vi "pathplan.vi"(8 "当前位置":dbl[](array[numeric]), 9 "目标位置（x,y）":dbl[](array[numeric]), 10 "障碍物Y":dbl[](array[numeric]), 11 "障碍物X":dbl[](array[numeric])) -> (1 "y":dbl[](array[numeric]), 2 "x":dbl[](array[numeric]))   [LabVIEW 2016]
uses:
  <vilib>/gmath/SpecialFunctions.llb/Factorial.vi
  <vilib>/imath/engines/lvmath2/RunTimeEngine/BuiltInFunctions/size/NIMS_I32Row=size(GRow).vi
  <instcachedir>/0/NIMS_I32Row=size(GRow)_E5C05C6B13124B29B774CC4F993D3C59.lvgen/NIMS_I32Row=size(GRow)_E5C05C6B13124B29B774CC4F993D3C59_000.vi
  <vilib>/imath/engines/lvmath2/RunTimeEngine/IndexRead/NIMS M(S,S).vi
  <instcachedir>/0/NIMS M(S,S)_AC51E74150A542F7991B9634C66F3096.lvgen/NIMS M(S,S)_AC51E74150A542F7991B9634C66F3096_002.vi
  <vilib>/imathl/engines/lvmath/Functions/Error Handling/Create Error.vi
  <vilib>/imath/engines/lvmath2/RunTimeEngine/IndexRead/NIMS V(S).vi
  <instcachedir>/0/NIMS V(S)_0488751826AF41519A22953C041130DC.lvgen/NIMS V(S)_0488751826AF41519A22953C041130DC_000.vi
  <vilib>/imath/engines/lvmath2/RunTimeEngine/IndexReplace/NIMS V(S)=S.vi
  <instcachedir>/0/NIMS V(S)=S_5B9D821375184D3582A2146CD1A04ED7.lvgen/NIMS V(S)=S_5B9D821375184D3582A2146CD1A04ED7_001.vi
  <vilib>/imath/engines/lvmath2/RunTimeEngine/ErrorHandling/NIMS_Create Error From Enums.vi
  <vilib>/imath/engines/lvmath2/RunTimeEngine/BuiltInFunctions/power/NIMS_power.vi
  <instcachedir>/0/NIMS_power_10DB0E02FC3E47EE88A20FD73927AD27.lvgen/NIMS_power_10DB0E02FC3E47EE88A20FD73927AD27_016.vi
  <instcachedir>/0/NIMS V(S)_0488751826AF41519A22953C041130DC.lvgen/NIMS V(S)_0488751826AF41519A22953C041130DC_003.vi
  <vilib>/imath/engines/lvmath2/RunTimeEngine/BuiltInFunctions/cos/NIMS_cos(C).vi
  <instcachedir>/0/NIMS_cos(C)_6CBFAE4528E34B94A77DA2891B495EBE.lvgen/NIMS_cos(C)_6CBFAE4528E34B94A77DA2891B495EBE_001.vi
  <vilib>/imath/engines/lvmath2/RunTimeEngine/BuiltInFunctions/abs/NIMS_abs(signed).vi
  <instcachedir>/0/NIMS_abs(signed)_C4FCB8E6058B49B797C7C8D53CA5F6EC.lvgen/NIMS_abs(signed)_C4FCB8E6058B49B797C7C8D53CA5F6EC_002.vi
  <vilib>/imath/engines/lvmath2/RunTimeEngine/RangeToken/NIMS_Range_R2 - Integer.vi
  <instcachedir>/0/NIMS_Range_R2 - Integer_416A044C4F024DBE8E97DA138CB3186F.lvgen/NIMS_Range_R2 - Integer_416A044C4F024DBE8E97DA138CB3186F_000.vi
  <vilib>/imath/engines/lvmath2/RunTimeEngine/CommandStatement/MC_CommandStatement_break.vi
  <vilib>/imath/engines/lvmath/Functions/Error Handling/MergeErrorsWrapper.vi
  <vilib>/imath/engines/lvmath2/RunTimeEngine/IndexReplace/NIMS M(S)=S.vi
  <instcachedir>/0/NIMS M(S)=S_9328EF344EC9443A8B5E4239F1A18A91.lvgen/NIMS M(S)=S_9328EF344EC9443A8B5E4239F1A18A91_001.vi
  <vilib>/imath/engines/lvmath2/RunTimeEngine/ArithmeticOperatorToken/NIMS_ArithmeticOperator_minus.vi
  <instcachedir>/0/NIMS_ArithmeticOperator_minus_DDDC508CE2F847AF862BE7DD2E3133BB.lvgen/NIMS_ArithmeticOperator_minus_DDDC508CE2F847AF862BE7DD2E3133BB_003.vi
  <vilib>/imath/engines/lvmath2/RunTimeEngine/BuiltInFunctions/norm/NIMS_norm(GV,DBL).vi
  <instcachedir>/0/NIMS_norm(GV,DBL)_AEE3258AE133461381C802EA81F1ACD5.lvgen/NIMS_norm(GV,DBL)_AEE3258AE133461381C802EA81F1ACD5_000.vi
  <vilib>/imath/engines/lvmath2/RunTimeEngine/IndexRead/NIMS M(S).vi
  <instcachedir>/0/NIMS M(S)_B826C018497E4940AE96BD27B540B6FB.lvgen/NIMS M(S)_B826C018497E4940AE96BD27B540B6FB_000.vi
  <vilib>/imath/engines/lvmath2/RunTimeEngine/IndexRead/NIMS V(V).vi
  <instcachedir>/0/NIMS V(V)_298D9CB7BFEB42B8BC8D9C3C28AE8C70.lvgen/NIMS V(V)_298D9CB7BFEB42B8BC8D9C3C28AE8C70_000.vi
  <vilib>/imath/engines/lvmath2/RunTimeSupport/NIMS_Get Scalar_w Error.vi
  <instcachedir>/0/NIMS_Get Scalar_w Error_B10CD3EFE684481FAA3AC86F54EE16C9.lvgen/NIMS_Get Scalar_w Error_B10CD3EFE684481FAA3AC86F54EE16C9_010.vi
  <vilib>/imath/engines/lvmath2/RunTimeEngine/MatrixToken/NIMS_MatrixToken_RV_RV.vi
  <instcachedir>/0/NIMS_MatrixToken_RV_RV_EF9D95F1EBB54EC7B599CEAAF2A767A1.lvgen/NIMS_MatrixToken_RV_RV_EF9D95F1EBB54EC7B599CEAAF2A767A1_002.vi
  <vilib>/imath/engines/lvmath2/RunTimeEngine/MatrixToken/NIMS_MatrixToken_M_RV.vi
  <instcachedir>/0/NIMS_MatrixToken_M_RV_FA7C223A39F54BCB827124D804A50E22.lvgen/NIMS_MatrixToken_M_RV_FA7C223A39F54BCB827124D804A50E22_001.vi
  <vilib>/imath/engines/lvmath2/RunTimeEngine/BuiltInFunctions/max/2 inputs/NIMS_max(RG,RG)-no size check.vi
  <instcachedir>/0/NIMS_max(RG,RG)-no size check_F871939977644B7683C1350DCCAD7557.lvgen/NIMS_max(RG,RG)-no size check_F871939977644B7683C1350DCCAD7557_000.vi
  <instcachedir>/0/NIMS M(S,S)_AC51E74150A542F7991B9634C66F3096.lvgen/NIMS M(S,S)_AC51E74150A542F7991B9634C66F3096_000.vi
  <vilib>/imath/engines/lvmath2/RunTimeEngine/BuiltInFunctions/min/2 inputs/NIMS_min(RG,RG)-no size check.vi
  <instcachedir>/0/NIMS_min(RG,RG)-no size check_7F67BAB91AFC452D9517D2EA1C8F5F88.lvgen/NIMS_min(RG,RG)-no size check_7F67BAB91AFC452D9517D2EA1C8F5F88_001.vi
  <instcachedir>/0/NIMS_abs(signed)_C4FCB8E6058B49B797C7C8D53CA5F6EC.lvgen/NIMS_abs(signed)_C4FCB8E6058B49B797C7C8D53CA5F6EC_000.vi
  <vilib>/imath/engines/lvmath2/RunTimeEngine/VariableToken/NIMS_VariableToken_CondDefined.vi
  <instcachedir>/0/NIMS_VariableToken_CondDefined_620A15720FCC4DA7863546285C12295E.lvgen/NIMS_VariableToken_CondDefined_620A15720FCC4DA7863546285C12295E_001.vi
  <vilib>/imath/engines/lvmath2/RunTimeEngine/BuiltInFunctions/size/NIMS_I32=size(GM,I32).vi
  <instcachedir>/0/NIMS_I32=size(GM,I32)_9B6975FE2A37478D9DF1A6A9597B9E6B.lvgen/NIMS_I32=size(GM,I32)_9B6975FE2A37478D9DF1A6A9597B9E6B_004.vi
  <vilib>/imath/engines/lvmath2/RunTimeEngine/NodeEndStatement/NIMS_NodeEndStatement_Output.vi
  <instcachedir>/0/NIMS_NodeEndStatement_Output_53EC0D466D134D7ABD903AC30B43404B.lvgen/NIMS_NodeEndStatement_Output_53EC0D466D134D7ABD903AC30B43404B_005.vi
  <vilib>/imath/engines/lvmath2/RunTimeEngine/ErrorHandling/NIMS_Finalize Error.vi
  <vilib>/gmath/NI_Gmath.lvlib
panel:
  out "?":cluster{"Data_x":dbl[], "Data_y":dbl[]}(graph)
  out "x/y":dbl[](array[numeric])
  out "?":cluster{"Data_x":dbl[], "Data_y":dbl[]}(graph)
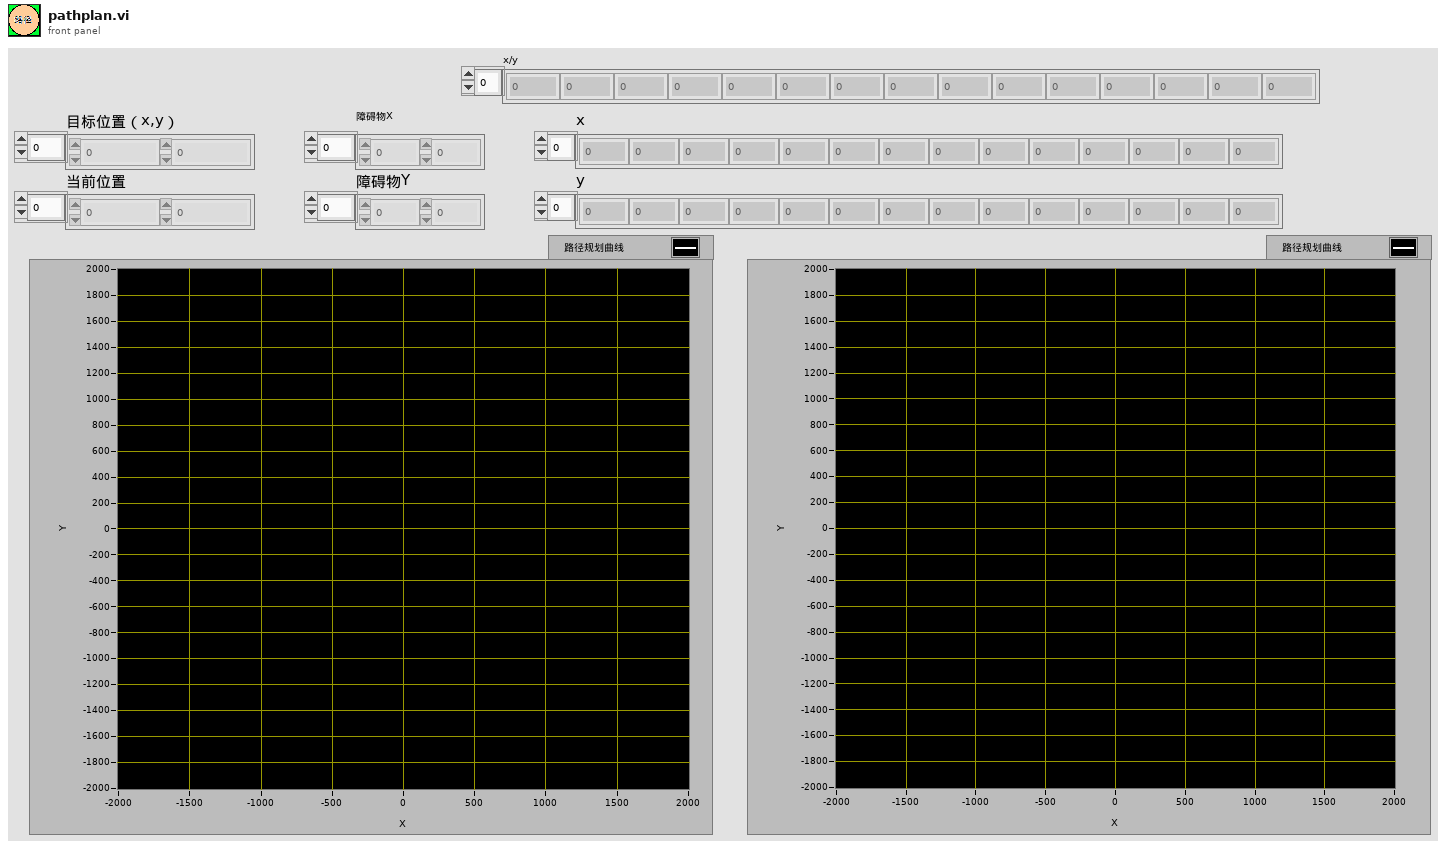
[diagram p1: front panel]
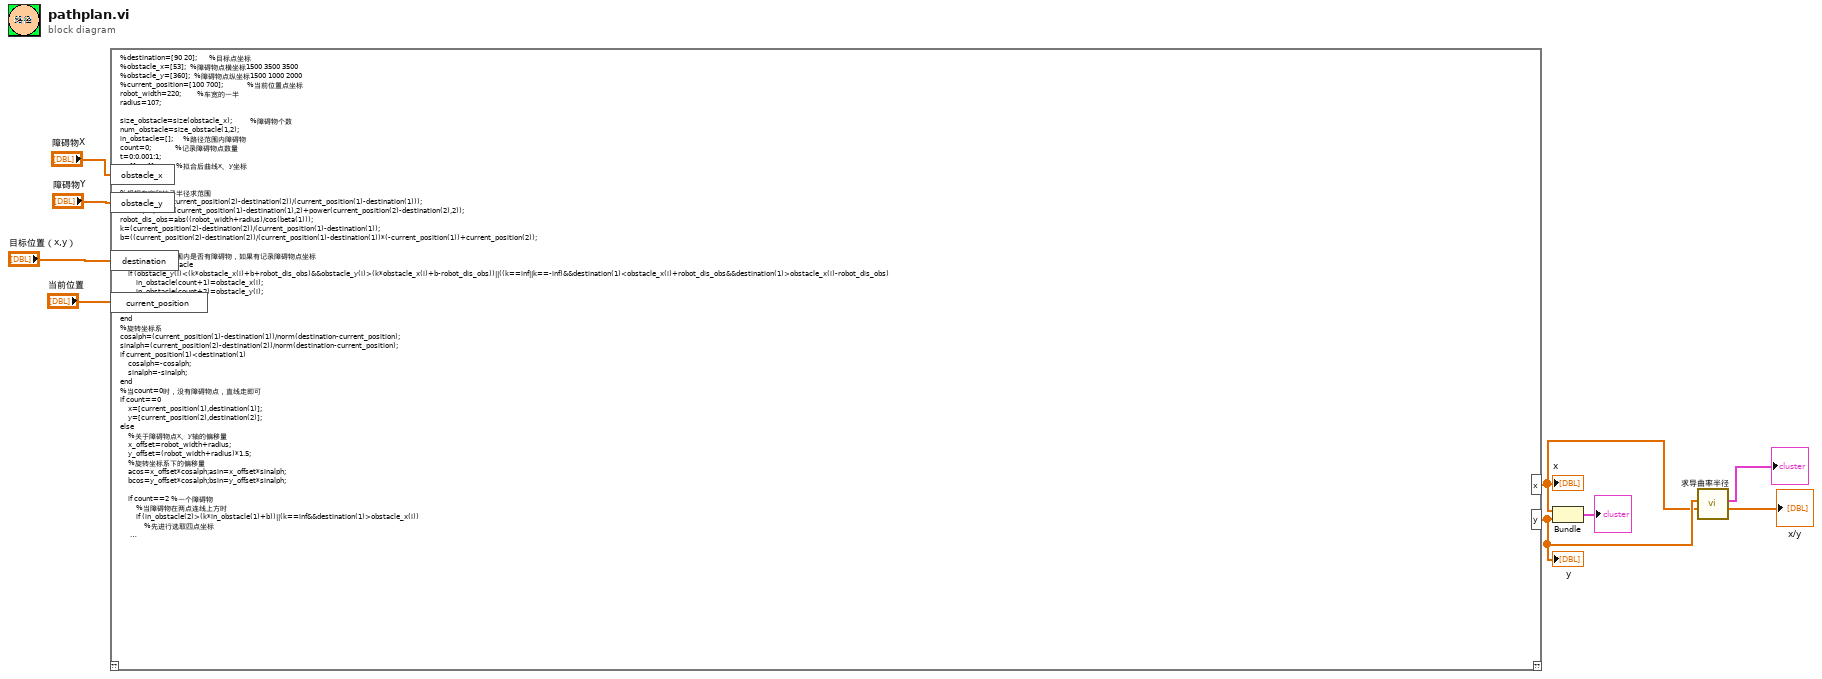
[diagram p0: block diagram]
diagram:
  n1 = mathscript code="%destination=[90 20];      %目标点坐标\n%obstacle_x=[53];  %障碍物点横坐标1500 3500 3500\n%obstacle_y=[360];  %障碍物点纵坐标1500 1000 2000\n%current_position=[100 700];            %当前位置点坐标\nrobot_width=220;        %车宽的一半\nradius=107;\n\nsize_obstacle=size(obstacle_x);         %障碍物个数\nnum_obstacle=size_obstacle(1,2);\nin_obstacle=[];     %路径范围内障碍物\ncount=0;            %记录障碍物点数量\nt=0:0.001:1;\nx=[];y=[];          %拟合后曲线x、y坐标\n\n\n%根据车宽和柱子半径求范围\nbeta(1)=atan((current_position(2)-destination(2))/(current_position(1)-destination(1)));\ndis=sqrt(power(current_position(1)-destination(1),2)+power(current_position(2)-destination(2),2));\nrobot_dis_obs=abs((robot_width+radius)/cos(beta(1)));\nk=(current_position(2)-destination(2))/(current_position(1)-destination(1));\nb=((current_position(2)-destination(2))/(current_position(1)-destination(1))*(-current_position(1))+current_position(2));\n\n%判断直行路径范围内是否有障碍物，如果有记录障碍物点坐标\nfor i=1:num_obstacle\n    if (obstacle_y(i)<(k*obstacle_x(i)+b+robot_dis_obs)&&obstacle_y(i)>(k*obstacle_x(i)+b-robot_dis_obs))||((k==inf||k==-inf)&&destination(1)<obstacle_x(i)+robot_dis_obs&&destination(1)>obstacle_x(i)-robot_dis_obs)\n        in_obstacle(count+1)=obstacle_x(i);\n        in_obstacle(count+2)=obstacle_y(i);\n        count=count+2;\n    end\nend\n%旋转坐标系\ncosalph=(current_position(1)-destination(1))/norm(destination-current_position);\nsinalph=(current_position(2)-destination(2))/norm(destination-current_position);\nif current_position(1)<destination(1)\n    cosalph=-cosalph;\n    sinalph=-sinalph;\nend\n%当count=0时，没有障碍物点，直线走即可\nif count==0\n    x=[current_position(1),destination(1)];\n    y=[current_position(2),destination(2)];\nelse\n    %关于障碍物点x、y轴的偏移量\n    x_offset=robot_width+radius;\n    y_offset=(robot_width+radius)*1.5;\n    %旋转坐标系下的偏移量\n    acos=x_offset*cosalph;asin=x_offset*sinalph;\n    bcos=y_offset*cosalph;bsin=y_offset*sinalph;\n    \n    if count==2 %一个障碍物\n        %当障碍物在两点连线上方时\n        if (in_obstacle(2)>(k*in_obstacle(1)+b))||(k==inf&&destination(1)>obstacle_x(i))\n            %先进行选取四点坐标\n            temp_position1=[in_obstacle(1)+acos+bsin,in_obstacle(2)+asin-bcos];\n            temp_position2=[in_obstacle(1)-acos+bsin,in_obstacle(2)-asin-bcos];\n            if current_position(1)>destination(1)\n                if temp_position1(1)>temp_position2(1)\n                    vertices=[current_position;temp_position1;temp_position2;destination]';\n                else\n                    vertices=[current_position;temp_position2;temp_position1;destination]';\n                end\n            else\n                if temp_position1(1)>temp_position2(1)\n                    vertices=[current_position;temp_position2;temp_position1;destination]';\n                else\n                    vertices=[current_position;temp_position1;temp_position2;destination]';\n                end\n            end\n            %检测两两坐标连线上是否会遇到障碍物\n            for i=1:num_obstacle\n                %待检测出的障碍物的横坐标应不等于已检测出障碍物点的横坐标，检测右边是否有障碍物\n                if (obstacle_x(i)~=in_obstacle(1))&&(obstacle_x(i)<max(current_position(1),destination(1)))&&(obstacle_y(i)<((vertices(2,2)-vertices(2,1))/(vertices(1,2)-vertices(1,1))*obstacle_x(i)+vertices(2,2)-(vertices(2,2)-vertices(2,1))/(vertices(1,2)-vertices(1,1))*vertices(1,2)+robot_dis_obs))&&(obstacle_y(i)>((vertices(2,2)-vertices(2,1))/(vertices(1,2)-vertices(1,1))*obstacle_x(i)+vertices(2,2)-(vertices(2,2)-vertices(2,1))/(vertices(1,2)-vertices(1,1))*vertices(1,2)-robot_dis_obs))\n                    in_obstacle(count+1)=obstacle_x(i);     %若有，记录下该障碍物点的横纵坐标，count加2\n                    in_obstacle(count+2)=obstacle_y(i);\n                    count=count+2;\n                    %检测左边是否有障碍物\n                elseif (obstacle_x(i)~=in_obstacle(1))&&(obstacle_x(i)>min(current_position(1),destination(1)))&&(obstacle_y(i)<((vertices(2,4)-vertices(2,3))/(vertices(1,4)-vertices(1,3))*obstacle_x(i)+vertices(2,4)-(vertices(2,4)-vertices(2,3))/(vertices(1,4)-vertices(1,3))*vertices(1,4)+robot_dis_obs))&&(obstacle_y(i)>((vertices(2,4)-vertices(2,3))/(vertices(1,4)-vertices(1,3))*obstacle_x(i)+vertices(2,4)-(vertices(2,4)-vertices(2,3))/(vertices(1,4)-vertices(1,3))*vertices(1,4)-robot_dis_obs))\n                    tempx=in_obstacle(1);\n                    tempy=in_obstacle(2);\n                    in_obstacle(1)=obstacle_x(i);\n                    in_obstacle(2)=obstacle_y(i);\n                    in_obstacle(3)=tempx;\n                    in_obstacle(4)=tempy;\n                    count=count+2;\n                end\n            end\n        else\n            temp_position1=[in_obstacle(1)+acos-bsin,in_obstacle(2)+asin+bcos];\n            temp_position2=[in_obstacle(1)-acos-bsin,in_obstacle(2)-asin+bcos];\n            if current_position(1)>destination(1)\n                if temp_position1(1)>temp_position2(1)\n                    vertices=[current_position;temp_position1;temp_position2;destination]';\n                else\n                    vertices=[current_position;temp_position2;temp_position1;destination]';\n                end\n            else\n                if temp_position1(1)>temp_position2(1)\n                    vertices=[current_position;temp_position2;temp_position1;destination]';\n                else\n                    vertices=[current_position;temp_position1;temp_position2;destination]';\n                end\n            end\n            for i=1:num_obstacle\n                if (obstacle_x(i)~=in_obstacle(1))&&(obstacle_x(i)<max(current_position(1),destination(1)))&&(obstacle_y(i)<((vertices(2,2)-vertices(2,1))/(vertices(1,2)-vertices(1,1))*obstacle_x(i)+vertices(2,2)-(vertices(2,2)-vertices(2,1))/(vertices(1,2)-vertices(1,1))*vertices(1,2)+robot_dis_obs))&&(obstacle_y(i)>((vertices(2,2)-vertices(2,1))/(vertices(1,2)-vertices(1,1))*obstacle_x(i)+vertices(2,2)-(vertices(2,2)-vertices(2,1))/(vertices(1,2)-vertices(1,1))*vertices(1,2)-robot_dis_obs))\n                    in_obstacle(count+1)=obstacle_x(i);\n                    in_obstacle(count+2)=obstacle_y(i);\n                    count=count+2;\n                    break;\n                elseif (obstacle_x(i)~=in_obstacle(1))&&(obstacle_x(i)>min(current_position(1),destination(1)))&&(obstacle_y(i)<((vertices(2,4)-vertices(2,3))/(vertices(1,4)-vertices(1,3))*obstacle_x(i)+vertices(2,4)-(vertices(2,4)-vertices(2,3))/(vertices(1,4)-vertices(1,3))*vertices(1,4)+robot_dis_obs))&&(obstacle_y(i)>((vertices(2,4)-vertices(2,3))/(vertices(1,4)-vertices(1,3))*obstacle_x(i)+vertices(2,4)-(vertices(2,4)-vertices(2,3))/(vertices(1,4)-vertices(1,3))*vertices(1,4)-robot_dis_obs))\n                    tempx=in_obstacle(1);\n                    tempy=in_obstacle(2);\n                    in_obstacle(1)=obstacle_x(i);\n                    in_obstacle(2)=obstacle_y(i);\n                    in_obstacle(3)=tempx;\n                    in_obstacle(4)=tempy;\n                    count=count+2;\n                    break;\n                end\n            end\n        end\n    end\n    if count==2\n    else\n        %当两个都在直线上方时\n        if (in_obstacle(2)>(k*in_obstacle(1)+b)||in_obstacle(2)==(k*in_obstacle(1)+b))&&(in_obstacle(4)>(k*in_obstacle(3)+b)||in_obstacle(4)==(k*in_obstacle(3)+b))\n            temp_position1=[in_obstacle(3)+acos+bsin,in_obstacle(4)+asin-bcos];\n            temp_position2=[in_obstacle(3)-acos+bsin,in_obstacle(4)-asin-bcos];\n            temp_position3=[in_obstacle(1)+acos+bsin,in_obstacle(2)+asin-bcos];\n            temp_position4=[in_obstacle(1)-acos+bsin,in_obstacle(2)-asin-bcos];\n            if abs(current_position(1)-in_obstacle(3))<abs(current_position(1)-in_obstacle(1))\n                if abs(current_position(1)-temp_position1(1))<abs(current_position(1)-temp_position2(1))\n                    temp1=temp_position1;\n                    temp2=temp_position2;\n                else\n                    temp1=temp_position2;\n                    temp2=temp_position1;\n                end\n                if abs(destination(1)-temp_position3(1))>abs(destination(1)-temp_position4(1))\n                    temp3=temp_position3;\n                    temp4=temp_position4;\n                else\n                    temp3=temp_position4;\n                    temp4=temp_position3;\n                end\n                vertices=[current_position;temp1;temp2;temp3;temp4;destination ]';\n            else\n                if abs(current_position(1)-temp_position3(1))<abs(current_position(1)-temp_position4(1))\n                    temp1=temp_position3;\n                    temp2=temp_position4;\n                else\n                    temp1=temp_position4;\n                    temp2=temp_position3;\n                end\n                if abs(destination(1)-temp_position1(1))>abs(destination(1)-temp_position2(1))\n                    temp3=temp_position1;\n                    temp4=temp_position2;\n                else\n                    temp3=temp_position2;\n                    temp4=temp_position1;\n                end\n                vertices=[current_position;temp1;temp2;temp3;temp4;destination ]';\n            end\n            %当右侧的在直线下方，左侧的在直线上方\n        elseif in_obstacle(2)<(k*in_obstacle(1)+b)&&in_obstacle(4)>(k*in_obstacle(3)+b)\n            y_offset=(robot_width+radius)*2;\n            bcos=y_offset*cosalph;bsin=y_offset*sinalph;\n            temp_position1=[in_obstacle(3)+acos+bsin,in_obstacle(4)+asin-bcos];\n            temp_position2=[in_obstacle(3)-acos+bsin,in_obstacle(4)-asin-bcos];\n            temp_position3=[in_obstacle(1)+acos-bsin,in_obstacle(2)+asin+bcos];\n            temp_position4=[in_obstacle(1)-acos-bsin,in_obstacle(2)-asin+bcos];\n            if abs(current_position(1)-in_obstacle(3))<abs(current_position(1)-in_obstacle(1))\n                if abs(current_position(1)-temp_position1(1))<abs(current_position(1)-temp_position2(1))\n                    temp1=temp_position1;\n                    temp2=temp_position2;\n                else\n                    temp1=temp_position2;\n                    temp2=temp_position1;\n                end\n                if abs(destination(1)-temp_position3(1))>abs(destination(1)-temp_position4(1))\n                    temp3=temp_position3;\n                    temp4=temp_position4;\n                else\n                    temp3=temp_position4;\n                    temp4=temp_position3;\n                end\n                vertices=[current_position;temp1;temp2;temp3;temp4;destination ]';\n            else\n                if abs(current_position(1)-temp_position3(1))<abs(current_position(1)-temp_position4(1))\n                    temp1=temp_position3;\n                    temp2=temp_position4;\n                else\n                    temp1=temp_position4;\n                    temp2=temp_position3;\n                end\n                if abs(destination(1)-temp_position1(1))>abs(destination(1)-temp_position2(1))\n                    temp3=temp_position1;\n                    temp4=temp_position2;\n                else\n                    temp3=temp_position2;\n                    temp4=temp_position1;\n                end\n                vertices=[current_position;temp1;temp2;temp3;temp4;destination ]';\n            end\n            %当右侧的在直线上方，左侧的在直线下方\n        elseif in_obstacle(2)>(k*in_obstacle(1)+b)&&in_obstacle(4)<(k*in_obstacle(3)+b)\n            y_offset=(robot_width+radius)*2;\n            bcos=y_offset*cosalph;bsin=y_offset*sinalph;\n            temp_position1=[in_obstacle(3)+acos-bsin,in_obstacle(4)+asin+bcos];\n            temp_position2=[in_obstacle(3)-acos-bsin,in_obstacle(4)-asin+bcos];\n            temp_position3=[in_obstacle(1)+acos+bsin,in_obstacle(2)+asin-bcos];\n            temp_position4=[in_obstacle(1)-acos+bsin,in_obstacle(2)-asin-bcos];\n            if abs(current_position(1)-in_obstacle(3))<abs(current_position(1)-in_obstacle(1))\n                if abs(current_position(1)-temp_position1(1))<abs(current_position(1)-temp_position2(1))\n                    temp1=temp_position1;\n                    temp2=temp_position2;\n                else\n                    temp1=temp_position2;\n                    temp2=temp_position1;\n                end\n                if abs(destination(1)-temp_position3(1))>abs(destination(1)-temp_position4(1))\n                    temp3=temp_position3;\n                    temp4=temp_position4;\n                else\n                    temp3=temp_position4;\n                    temp4=temp_position3;\n                end\n                vertices=[current_position;temp1;temp2;temp3;temp4;destination ]';\n            else\n                if abs(current_position(1)-temp_position3(1))<abs(current_position(1)-temp_position4(1))\n                    temp1=temp_position3;\n                    temp2=temp_position4;\n                else\n                    temp1=temp_position4;\n                    temp2=temp_position3;\n                end\n                if abs(destination(1)-temp_position1(1))>abs(destination(1)-temp_position2(1))\n                    temp3=temp_position1;\n                    temp4=temp_position2;\n                else\n                    temp3=temp_position2;\n                    temp4=temp_position1;\n                end\n                vertices=[current_position;temp1;temp2;temp3;temp4;destination ]';\n            end\n        else%当两点都在直线下方时\n            temp_position1=[in_obstacle(3)+acos-bsin,in_obstacle(4)+asin+bcos];\n            temp_position2=[in_obstacle(3)-acos-bsin,in_obstacle(4)-asin+bcos];\n            temp_position3=[in_obstacle(1)+acos-bsin,in_obstacle(2)+asin+bcos];\n            temp_position4=[in_obstacle(1)-acos-bsin,in_obstacle(2)-asin+bcos];\n            if abs(current_position(1)-in_obstacle(3))<abs(current_position(1)-in_obstacle(1))\n                if abs(current_position(1)-temp_position1(1))<abs(current_position(1)-temp_position2(1))\n                    temp1=temp_position1;\n                    temp2=temp_position2;\n                else\n                    temp1=temp_position2;\n                    temp2=temp_position1;\n                end\n                if abs(destination(1)-temp_position3(1))>abs(destination(1)-temp_position4(1))\n                    temp3=temp_position3;\n                    temp4=temp_position4;\n                else\n                    temp3=temp_position4;\n                    temp4=temp_position3;\n                end\n                vertices=[current_position;temp1;temp2;temp3;temp4;destination ]';\n            else\n                if abs(current_position(1)-temp_position3(1))<abs(current_position(1)-temp_position4(1))\n                    temp1=temp_position3;\n                    temp2=temp_position4;\n                else\n                    temp1=temp_position4;\n                    temp2=temp_position3;\n                end\n                if abs(destination(1)-temp_position1(1))>abs(destination(1)-temp_position2(1))\n                    temp3=temp_position1;\n                    temp4=temp_position2;\n                else\n                    temp3=temp_position2;\n                    temp4=temp_position1;\n                end\n                vertices=[current_position;temp1;temp2;temp3;temp4;destination ]';\n            end\n        end\n    end\n    %贝塞尔曲线拟合\n    NumPoint=size(vertices,2)-1;\n    x=(1-t).^(NumPoint)*vertices(1,1);\n    y=(1-t).^(NumPoint)*vertices(2,1);\n    for j=1:NumPoint\n        w=factorial(NumPoint)/(factorial(j)*factorial(NumPoint-j))*(1-t).^(NumPoint-j).*t.^(j);\n        x=x+w*vertices(1,j+1);\n        y=y+w*vertices(2,j+1);\n    end\n\nend"("destination"="目标位置（x,y）", "obstacle_x"="障碍物X", "obstacle_y"="障碍物Y", "current_position"="当前位置") -> ("x"=w3:dbl[], "y"=w4:dbl[])  [unwired: 1 in, 1 out]
  "x" <- w3
  "y" <- w4
  n2 = Bundle("x"=w3, "y"=w4) -> (→"?":cluster{"x":dbl[], "y":dbl[]})  [unwired: 1 in]
  n3 = call "求导曲率半径.vi"("x"=w3, "y"=w4) -> ("x/y"=→"x/y":dbl[], 2:→"?":cluster{"Data_x":dbl[], "Data_y":dbl[]})  [unwired: 8 in]
